vi "opencvSegmentSingle.vi"(6 "maxYInStack":dbl, 7 "maxXInStack":dbl, 8 "ImgIn":u16[][](array[numeric])) -> (0 "NeuronN[last frame]":u16, 1 "maxY":dbl, 2 "NeuronXY[last frame]":u16[](array[numeric]), 4 "maxX":dbl)   [LabVIEW 2017]
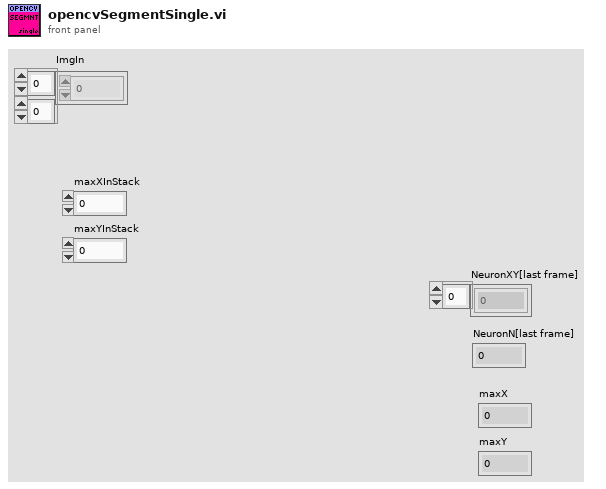
[diagram p1: front panel]
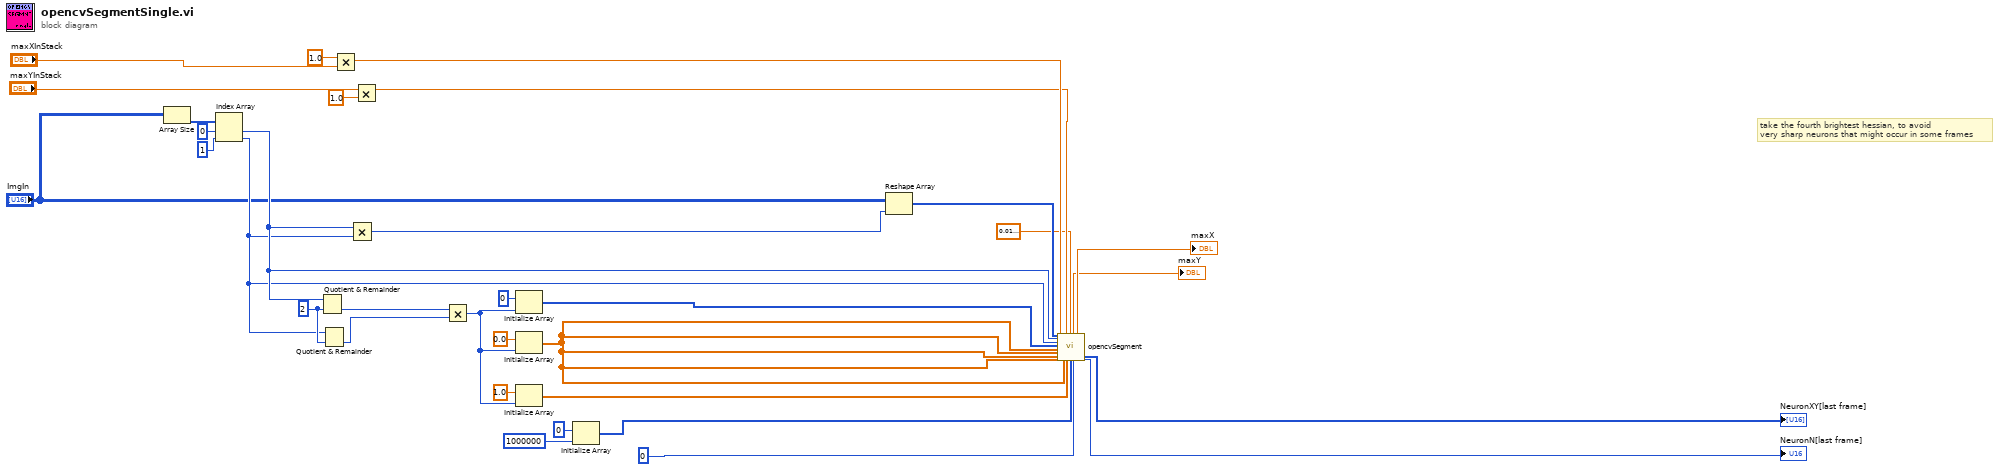
[diagram p0: block diagram]
diagram:
  w24 = 2 ("y")
  # "take the fourth brightest hessian, to avoid\nvery sharp neurons that might occur in some frames"
  n1 = Array Size(array="ImgIn") -> (size(s)=w33:i32[])
  n2 = Index Array(array=w33, index #1=0 ("index"), index #2=1 ("index")) -> (element #1=w22:i32, element #2=w21:i32)
  n3 = Quotient & Remainder(x=w22, y=w24) -> (floor(x/y)=w19:i32)  [unwired: 1 out]
  n4 = Quotient & Remainder(x=w21, y=w24) -> (floor(x/y)=w18:i32)  [unwired: 1 out]
  n5 = Multiply(x=1.0, y="maxXInStack") -> (x*y=w13:dbl)
  n6 = Multiply(x=w22, y=w21) -> (x*y=w20:i32)
  n7 = Multiply(x="maxYInStack", y=1.0) -> (x*y=w11:dbl)
  n8 = Multiply(x=w19, y=w18) -> (x*y=w23:i32)
  n9 = Initialize Array(u16 0 ("element"), w23) -> (w29:u16[])
  n10 = Initialize Array(sgl 0.0 ("element"), w23) -> (w9:sgl[])
  n11 = Initialize Array(sgl 1.0 ("element"), w23) -> (w28:sgl[])
  n12 = Initialize Array(u16 0 ("element"), 1000000 ("dimension size")) -> (w7:u16[])
  n13 = Reshape Array("ImgIn", w20) -> (w4:u16[])
  n14 = call "opencvSegment.vi"("ImgIn"=w4, "sizex"=w22, "sizey"=w21, "ArrA"=w29, "ArrB"=w9, "ArrBX"=w9, "ArrBY"=w9, "ArrBth"=w9, "maxXInStack"=w13, "ArrBdil"=w9, "maxYInStack"=w11, "ArrUno"=w28, "threshold"=sgl 0.02, "NeuronXY"=w7, "NeuronN"=u16 0) -> ("maxY"=→"maxY":dbl, "maxX"=→"maxX":dbl, "NeuronXY Out"=→"NeuronXY[last frame]":u16[], "NeuronN Out"=→"NeuronN[last frame]":u16)  [unwired: 2 in, 7 out]
